vi "73XX Motion Controller Main Page.vi"(8 "error in (no error)":errorcluster, 11 "Node Ptr":T4 format="%.0x") -> (0 "error out":errorcluster)   [LabVIEW 2010, in "73XX Motion Controller Custom Device.lvlib"]
uses:
  73XX Motion Controller Custom Device.lvlib
  <vilib>/NI VeriStand/Custom Device API/Custom Device Item Ref.ctl
  <vilib>/Motion/FlexMotion/CustomControls/CustomControls.llb/AxisOrVectorSpaceControl To Control.flx
  <vilib>/NI VeriStand/Custom Device API/Custom Device Channel.ctl
  <vilib>/NI VeriStand/Custom Device API/Custom Device Channel Type.ctl
  <vilib>/NI VeriStand/Custom Device API/Get Item Property (U16).vi
  <vilib>/NI VeriStand/Custom Device API/Set Item Property (U16).vi
  <vilib>/NI Veristand/Custom Device API/Custom Device API.lvlib
panel:
  in  "Operation Mode":T1(ring)
  in  "Axis or Vector Space":T2=1 items=["Axis Control"=0, "Axis 1"=1, "Axis 2"=2, "Axis 3"=3, "Axis 4"=4, "Axis 5"=5, "Axis 6"=6, "Axis 7"=7, "Axis 8"=8, "Vector Space Control"=16, "Vector Space 1"=17, "Vector Space 2"=18, "Vector Space 3"=19, "Vector Space 4"=20]
  in  "Board ID":T3=1 min=1 max=32 step=1
  in  "Header":cluster{"Section Name":string}={"Section Name"="Custom Device Item Settings"}
  in  "Description":string
  in  "Name":string
  in  "Delete":bool
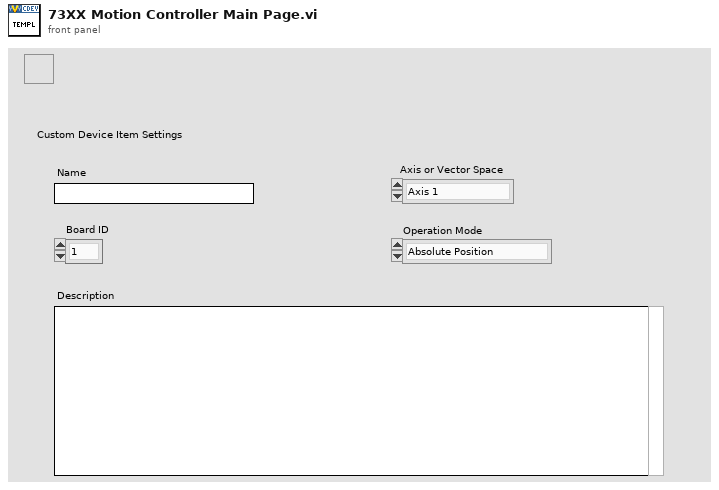
[diagram p1: front panel]
types:
  T1 = enum16{"Absolute Position", "Relative Position", "Velocity"}
  T2 = typedef "AxisOrVectorSpaceControl To Control.flx" = u16
  T3 = typedef "Board Id" = u8
  T4 = typedef "Custom Device API.lvlib/Custom Device Item Ref.ctl" = u64
  T5 = typedef "Custom Device API.lvlib/Custom Device Item Info.ctl" = cluster{"Name":string, "Is Channel":bool, "GUID":string}
  T6 = typedef "Custom Device API.lvlib/Custom Device Channel.ctl" = cluster{"Type":T7, "Units":string, "Default Value":dbl, "Faultable":bool, "Scalable":bool}
  T7 = typedef "Custom Device API.lvlib/Custom Device Channel Type.ctl" = enum16{"Input", "Output"}
  T8 = typedef "Custom Device API.lvlib/Custom Device Commands.ctl" = enum16{"Default", "Item renamed", "Shutdown", "Dynamic button pressed"}
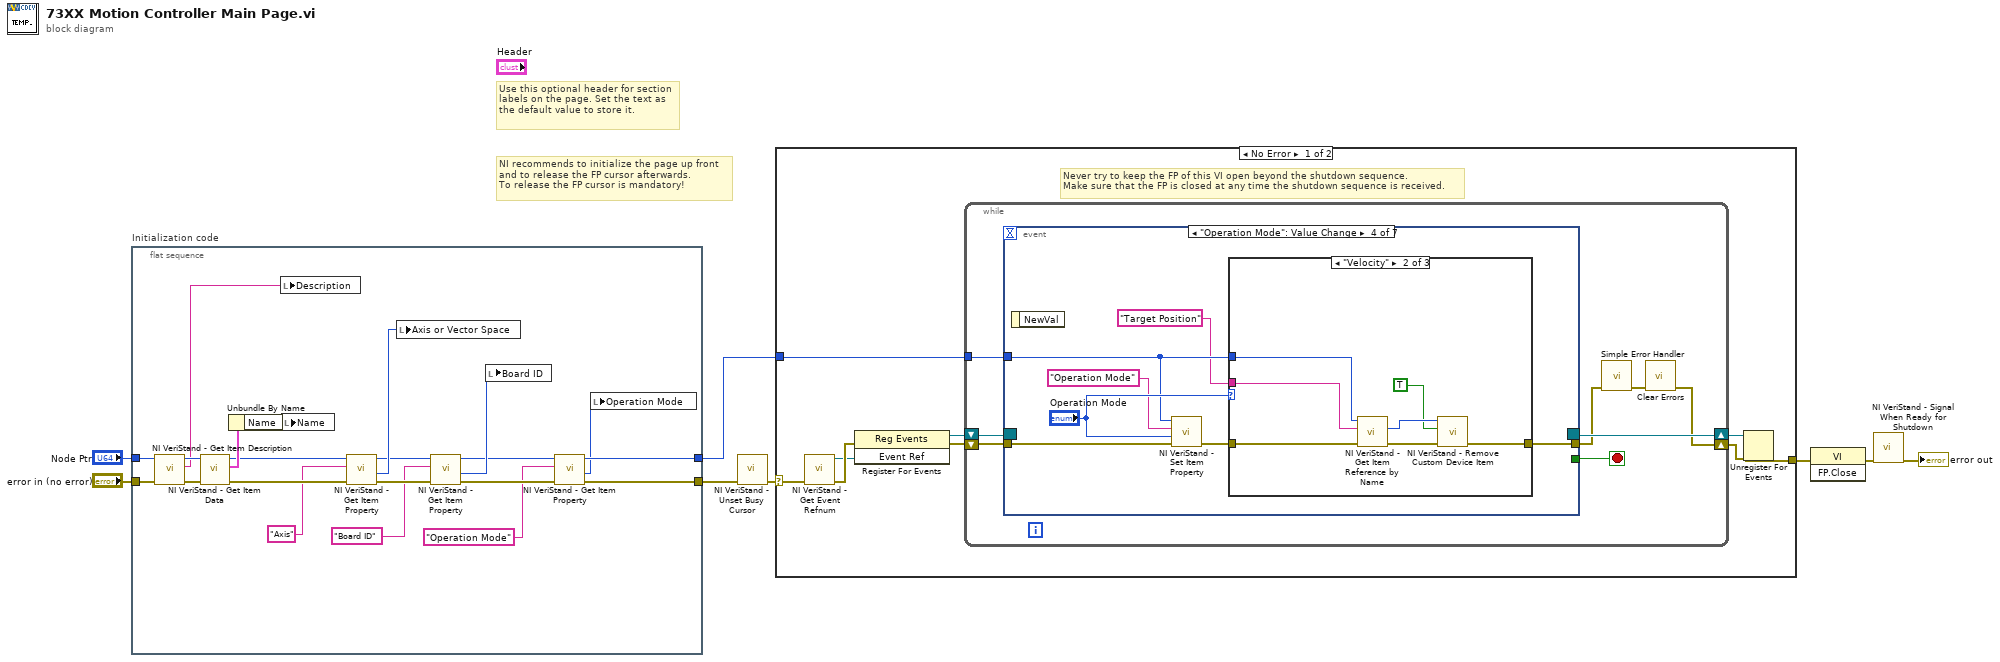
[diagram p0: block diagram]
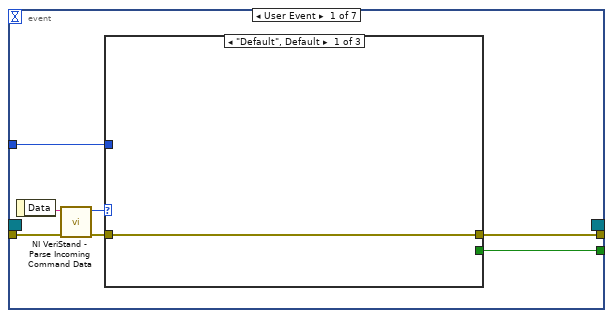
[diagram p2: hidden frame]
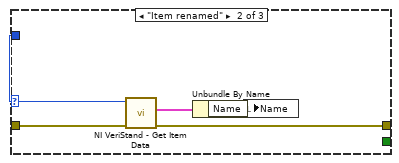
[diagram p3: hidden frame]
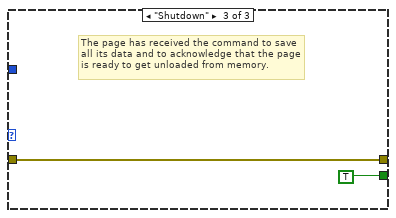
[diagram p4: hidden frame]
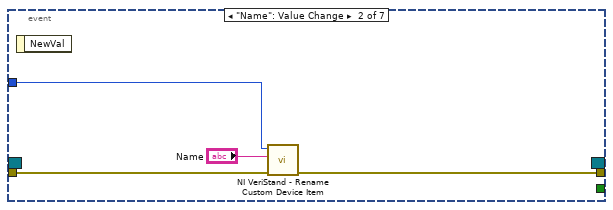
[diagram p5: hidden frame]
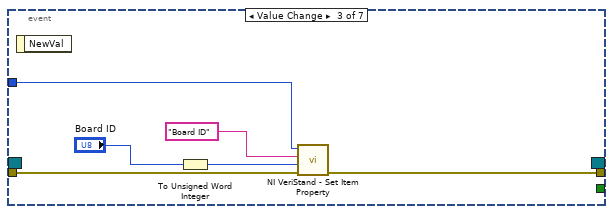
[diagram p6: hidden frame]
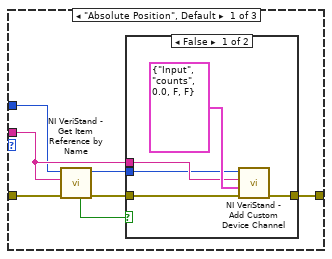
[diagram p7: hidden frame]
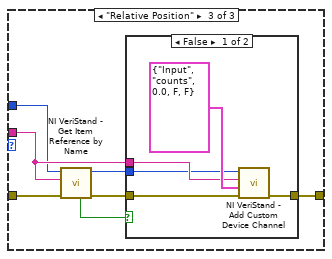
[diagram p9: hidden frame]
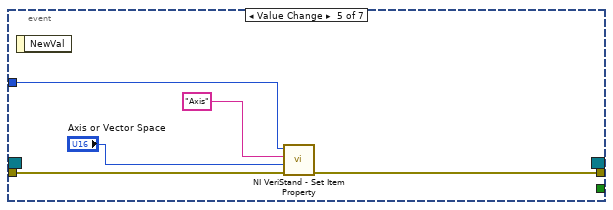
[diagram p11: hidden frame]
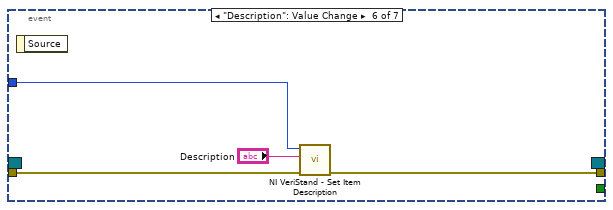
[diagram p12: hidden frame]
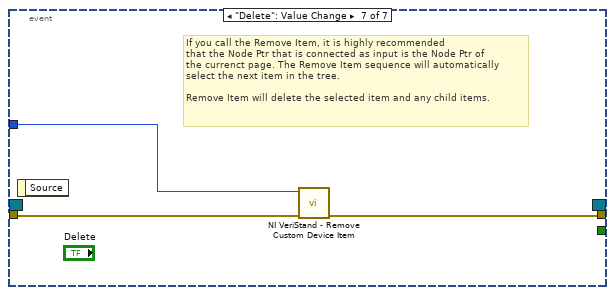
[diagram p13: hidden frame]
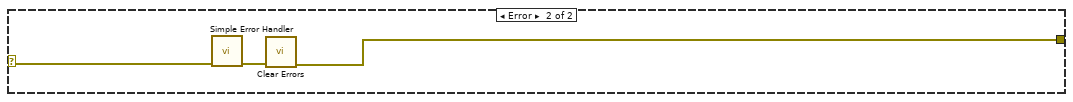
[diagram p14: hidden frame]
diagram:
  # "Use this optional header for section labels on the page. Set the text as the default value to store it."
  # "NI recommends to initialize the page up front\nand to release the FP cursor afterwards.\nTo release the FP cursor is mandatory!"
  n1 = flat-sequence "Initialization code" {
    tunnel: "error in (no error)" -> [w28]
    tunnel: "Node Ptr" -> [w27]
    tunnel: [w10] -> w4
    tunnel: [w11] -> w1
    frame #0 {
      n2 = call <vilib>:"NI VeriStand - Get Item Description.vi"("error in (no error)"=w28, "Item Ref in"=w27) -> ("error out"=w25:errorcluster, "Description"=w26:string, "Item Ref out"=w29:T4)  [unwired: 7 out]
      n3 = call <vilib>:"NI VeriStand - Get Item Data.vi"("error in (no error)"=w25, "Item Ref in"=w29) -> ("error out"=w22:errorcluster, "Item Info"=w24:T5, "Item Ref out"=w21:T4)  [unwired: 7 out]
      n4 = Unbundle By Name(w24) -> ("Name"=w23:string)
      n5 = local write "Description"(w26) -> ()
      n6 = local write "Name"(w23) -> ()
      n7 = call-poly <vilib>:"NI VeriStand - Get Item Property.vi"("error in (no error)"=w22, "Property Name"="Axis", "Item Ref in"=w21) -> ("error out"=w18:errorcluster, "Value"=w19:u16, "Item Ref out"=w17:T4)  [unwired: 5 in, 1 out]
      n8 = local write "Axis or Vector Space"(w19) -> ()
      n9 = call-poly <vilib>:"NI VeriStand - Get Item Property.vi"("error in (no error)"=w18, "Property Name"="Board ID", "Item Ref in"=w17) -> ("error out"=w14:errorcluster, "Value"=w16:u16, "Item Ref out"=w13:T4)  [unwired: 5 in, 1 out]
      n10 = local write "Board ID"(w16) -> ()
      n11 = call-poly <vilib>:"NI VeriStand - Get Item Property.vi"("error in (no error)"=w14, "Property Name"="Operation Mode", "Item Ref in"=w13) -> ("error out"=w10:errorcluster, "Value"=w9:u16, "Item Ref out"=w11:T4)  [unwired: 5 in, 1 out]
      n12 = local write "Operation Mode"(w9) -> ()
    }
  }
  n13 = call <vilib>:"NI VeriStand - Unset Busy Cursor.vi"("error in (no error)"=w4) -> ("error out"=w3:errorcluster)  [unwired: 10 out]
  n14 = case shown="No Error" w3 {
    selector: w3 -> [w30 w126]
    tunnel: [w35 w124] -> w8
    tunnel: w1 -> [w31 _]
    frame No Error {
      # "Never try to keep the FP of this VI open beyond the shutdown sequence.\nMake sure that the FP is closed at any time the shutdown sequence is received."
      n15 = call <vilib>:"NI VeriStand - Get Event Refnum.vi"("error in (no error)"=w30) -> ("error out"=w38:errorcluster, "Event Ref"=w34:refnum<user-event>)  [unwired: 9 out]
      n16 = register-events(error in=w38, w34) -> (reference out=w32:refnum<event-registration>, error out=w33:errorcluster)  [unwired: 1 in]
      n17 = while {
        tunnel: w31 -> [w42]
        shift-right: [w39] -> w36
        shift-left: w33 -> [w45]
        shift-right: [w46] -> w37
        shift-left: w32 -> [w44]
        stop <- w43 stop-if-true
        n18 = event shown="[3] \"Operation Mode\": Value Change" {
          selector: w44 -> [_ _ _ _ _ _ _]
          dyn-events: [_ _ _ _ _ _ _] -> w46
          timeout: _ -> [_ _ _ _ _ _ _]
          tunnel: w45 -> [w53 w65 w71 w78 w116 w119 w123]
          tunnel: [w49 _ _ _ _ _ _] -> w43
          tunnel: [w48 w64 w68 w73 w112 w118 w122] -> w41
          tunnel: w42 -> [w47 w63 w70 w74 w115 w120 w121]
          event User Event {
            n19 = event-data() -> ("Data"=w52:string)  [unwired: 1 out]
            n20 = call <vilib>:"NI VeriStand - Parse Incoming Command Data.vi"("error in (no error)"=w53, "Data"=w52) -> ("error out"=w51:errorcluster, "Action"=w50:T8)  [unwired: 8 out]
            n21 = case shown="\"Default\", Default" w50 {
              tunnel: w51 -> [w54 w59 w60]
              tunnel: [_ _ TRUE] -> w49
              tunnel: [w54 w56 w60] -> w48
              tunnel: w47 -> [_ w58 _]
              frame "Default", Default {
              }
              frame "Item renamed" {
                n22 = call <vilib>:"NI VeriStand - Get Item Data.vi"("error in (no error)"=w59, "Item Ref in"=w58) -> ("error out"=w56:errorcluster, "Item Info"=w57:T5)  [unwired: 8 out]
                n23 = Unbundle By Name(w57) -> ("Name"=w55:string)
                n24 = local write "Name"(w55) -> ()
              }
              frame "Shutdown" {
                # "The page has received the command to save all its data and to acknowledge that the page is ready to get unloaded from memory."
              }
            }
          }
          event "Name": Value Change {
            n25 = event-data() -> ()  [unwired: 2 out]
            n26 = call <vilib>:"NI VeriStand - Rename Custom Device Item.vi"("error in (no error)"=w65, "New Name"="Name", "Item Ref in"=w63) -> ("error out"=w64:errorcluster)  [unwired: 8 out]
          }
          event Value Change {
            n27 = event-data() -> ()  [unwired: 2 out]
            n28 = To Unsigned Word Integer(number="Board ID") -> (unsigned 16bit integer=w66:u16)
            n29 = call-poly <vilib>:"NI VeriStand - Set Item Property.vi"("error in (no error)"=w71, "Value"=w66, "Property Name"="Board ID", "Item Ref in"=w70) -> ("error out"=w68:errorcluster)  [unwired: 5 in, 2 out]
          }
          event "Operation Mode": Value Change {
            n30 = event-data() -> ()  [unwired: 2 out]
            n31 = call-poly <vilib>:"NI VeriStand - Set Item Property.vi"("error in (no error)"=w78, "Value"="Operation Mode", "Property Name"="Operation Mode", "Item Ref in"=w74) -> ("error out"=w76:errorcluster)  [unwired: 5 in, 2 out]
            n32 = case shown="\"Velocity\"" "Operation Mode" {
              tunnel: w76 -> [w85 w98 w105]
              tunnel: w74 -> [w80 w97 w100]
              tunnel: [w81 w95 w101] -> w73
              tunnel: "Target Position" ("Property Name") -> [w82 w92 w102]
              frame "Absolute Position", Default {
                n33 = call <vilib>:"NI VeriStand - Get Item Reference by Name.vi"("error in (no error)"=w85, "Item Name"=w82, "Parent Ref in"=w80) -> ("error out"=w83:errorcluster, "Parent Ref out"=w79:T4, "Found"=w84:bool)  [unwired: 5 in, 1 out]
                n34 = case shown="False" w84 {
                  tunnel: w83 -> [w89 w91]
                  tunnel: w82 -> [w88 _]
                  tunnel: [w87 w91] -> w81
                  tunnel: w79 -> [w86 _]
                  frame False {
                    n35 = call <vilib>:"NI VeriStand - Add Custom Device Channel.vi"("error in (no error)"=w89, "Channel"=T6 {"Type"=enum."Input", "Units"="counts", "Default Value"=0.0, "Faultable"=FALSE, "Scalable"=FALSE}, "Channel Name"=w88, "Parent Ref in"=w86) -> ("error out"=w87:errorcluster)  [unwired: 4 in, 3 out]
                  }
                  frame True {
                  }
                }
              }
              frame "Velocity" {
                n36 = call <vilib>:"NI VeriStand - Get Item Reference by Name.vi"("error in (no error)"=w98, "Item Name"=w92, "Parent Ref in"=w97) -> ("error out"=w96:errorcluster, "Item Ref"=w94:T4)  [unwired: 5 in, 2 out]
                n37 = call <vilib>:"NI VeriStand - Remove Custom Device Item.vi"("error in (no error)"=w96, "Force Delete (F)"=TRUE, "Item Ref in"=w94) -> ("error out"=w95:errorcluster)  [unwired: 8 out]
              }
              frame "Relative Position" {
                n38 = call <vilib>:"NI VeriStand - Get Item Reference by Name.vi"("error in (no error)"=w105, "Item Name"=w102, "Parent Ref in"=w100) -> ("error out"=w103:errorcluster, "Parent Ref out"=w99:T4, "Found"=w104:bool)  [unwired: 5 in, 1 out]
                n39 = case shown="False" w104 {
                  tunnel: w103 -> [w109 w111]
                  tunnel: w102 -> [w108 _]
                  tunnel: [w107 w111] -> w101
                  tunnel: w99 -> [w106 _]
                  frame False {
                    n40 = call <vilib>:"NI VeriStand - Add Custom Device Channel.vi"("error in (no error)"=w109, "Channel"=T6 {"Type"=enum."Input", "Units"="counts", "Default Value"=0.0, "Faultable"=FALSE, "Scalable"=FALSE}, "Channel Name"=w108, "Parent Ref in"=w106) -> ("error out"=w107:errorcluster)  [unwired: 4 in, 3 out]
                  }
                  frame True {
                  }
                }
              }
            }
          }
          event Value Change {
            n41 = event-data() -> ()  [unwired: 2 out]
            n42 = call-poly <vilib>:"NI VeriStand - Set Item Property.vi"("error in (no error)"=w116, "Value"="Axis or Vector Space", "Property Name"="Axis", "Item Ref in"=w115) -> ("error out"=w112:errorcluster)  [unwired: 5 in, 2 out]
          }
          event "Description": Value Change {
            n43 = event-data() -> ()  [unwired: 2 out]
            n44 = call <vilib>:"NI VeriStand - Set Item Description.vi"("error in (no error)"=w119, "Description"="Description", "Item Ref in"=w120) -> ("error out"=w118:errorcluster)  [unwired: 8 out]
          }
          event "Delete": Value Change {
            # "If you call the Remove Item, it is highly recommended\nthat the Node Ptr that is connected as input is the Node Ptr of\nthe currenct page. The Remove Item sequence will automatically\nselect the next item in the tree.\n\nRemove Item will delete the selected item and any child items."
            n45 = event-data() -> ()  [unwired: 2 out]
            n46 = call <vilib>:"NI VeriStand - Remove Custom Device Item.vi"("error in (no error)"=w123, "Item Ref in"=w121) -> ("error out"=w122:errorcluster)  [unwired: 1 in, 8 out]
          }
        }
        n47 = call <vilib>:"Simple Error Handler.vi"("error in (no error)"=w41) -> ("error out"=w40:errorcluster)  [unwired: 1 in, 7 out]
        n48 = call <vilib>:"Clear Errors.vi"("error in (no error)"=w40) -> ("error out"=w39:errorcluster)  [unwired: 6 out]
      }
      n49 = Unregister For Events(event registration refnum=w37, error in=w36) -> (error out=w35:errorcluster)
    }
    frame Error {
      n50 = call <vilib>:"Simple Error Handler.vi"("error in (no error)"=w126) -> ("error out"=w125:errorcluster)  [unwired: 1 in, 7 out]
      n51 = call <vilib>:"Clear Errors.vi"("error in (no error)"=w125) -> ("error out"=w124:errorcluster)  [unwired: 6 out]
    }
  }
  n52 = invoke class="VI" method="FP.Close"(error in=w8) -> (error out=w7:errorcluster)  [unwired: 2 in, 2 out]
  n53 = call <vilib>:"NI VeriStand - Signal When Ready for Shutdown.vi"("error in (no error)"=w7) -> ("error out"=→"error out":errorcluster)  [unwired: 10 out]
